vi "PB_Cburn_ESR.vi"(5 "# freq points":i32=61, 7 "# scans before track":i32=50, 11 "ESR Parameters":T1={"Window 1 time (s)"=0.012, "Window 2 time (s)"=5e-06, "Window 3 time (s) "=0.02, "Window 4 time (s)"=5e-07, "Window 4 channels"=[TRUE, FALSE, FALSE, TRUE], "Window 3 channels"=[TRUE, FALSE, TRUE, TRUE], "Window 2 channels"=[TRUE, FALSE, FALSE, TRUE], "Window 1 channels"=[TRUE, TRUE, FALSE, TRUE], "Path to ESR Burner"=path "C:/Users/Loncar/Desktop/ESR VIs - Srujan/Sam Kim/PB/ESRFreq.exe"}) -> ()   [LabVIEW 2012]
uses:
  ESR Window Parameters.ctl
panel:
  out "String":string
  # "MW freq step\ndwell time"
  # "MW freq step"
  # "Wait"
  # "Fluorescence\ncounting"
  # "Ctr sample clk"
  # "Wait"
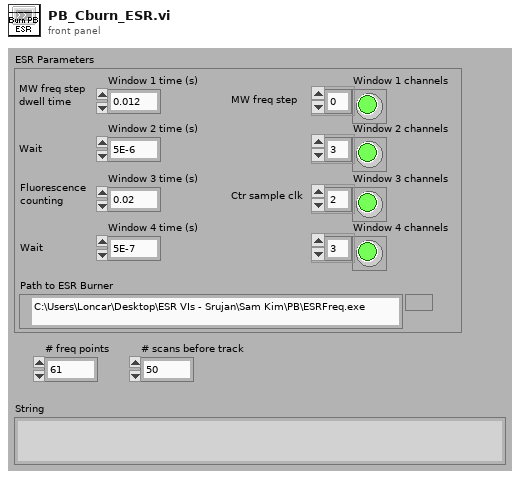
[diagram p1: front panel]
types:
  T1 = typedef "ESR Window Parameters.ctl" = cluster{"Window 1 time (s)":dbl, "Window 2 time (s)":dbl, "Window 3 time (s) ":dbl, "Window 4 time (s)":dbl, "Window 4 channels":bool[], "Window 3 channels":bool[], "Window 2 channels":bool[], "Window 1 channels":bool[], "Path to ESR Burner":path}
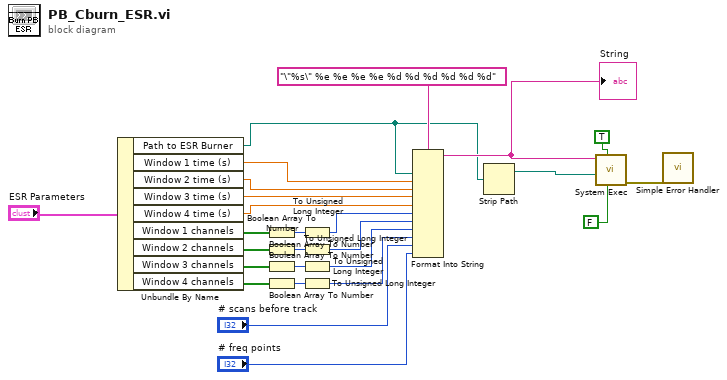
[diagram p0: block diagram]
diagram:
  n1 = Unbundle By Name("ESR Parameters") -> ("Path to ESR Burner"=w2:path, "Window 1 time (s)"=w10:dbl, "Window 2 time (s)"=w9:dbl, "Window 3 time (s)"=w8:dbl, "Window 4 time (s)"=w7:dbl, "Window 1 channels"=w6:bool[], "Window 2 channels"=w5:bool[], "Window 3 channels"=w4:bool[], "Window 4 channels"=w3:bool[])
  n2 = Boolean Array To Number(Boolean array=w6) -> (number=w23:u32)
  n3 = Boolean Array To Number(Boolean array=w5) -> (number=w22:u32)
  n4 = Boolean Array To Number(Boolean array=w4) -> (number=w21:u32)
  n5 = Boolean Array To Number(Boolean array=w3) -> (number=w20:u32)
  n6 = To Unsigned Long Integer(number=w23) -> (unsigned 32bit integer=w19:u32)
  n7 = To Unsigned Long Integer(number=w22) -> (unsigned 32bit integer=w18:u32)
  n8 = To Unsigned Long Integer(number=w21) -> (unsigned 32bit integer=w17:u32)
  n9 = To Unsigned Long Integer(number=w20) -> (unsigned 32bit integer=w16:u32)
  n10 = Format Into String(format string="\"%s\" %e %e %e %e %d %d %d %d %d %d", w2, w10, w9, w8, w7, w19, w18, w17, w16, "# scans before track", "# freq points") -> (resulting string=w12:string)  [unwired: 2 in, 1 out]
  "String" <- w12
  n11 = Strip Path(path=w2) -> (stripped path=w26:path)  [unwired: 1 out]
  n12 = call <vilib>:"System Exec.vi"("run minimized? (F)"=FALSE ("Wait until done"), "wait until completion? (T)"=TRUE ("Wait until done"), "working directory"=w26, "command line"=w12) -> ("error out"=w11:errorcluster)  [unwired: 4 in, 3 out]
  n13 = call <vilib>:"Simple Error Handler.vi"("error in (no error)"=w11) -> ()  [unwired: 4 in, 5 out]
